vi "Get Caraya Library Information.vi"() -> (1 "Library Info":T1, 2 "Caraya Library Path":path, 3 "reserved":refnum<class>)   [LabVIEW 2013, in "Caraya.lvlib"]
uses:
  Caraya.lvlib
  Caraya Library Info.ctl
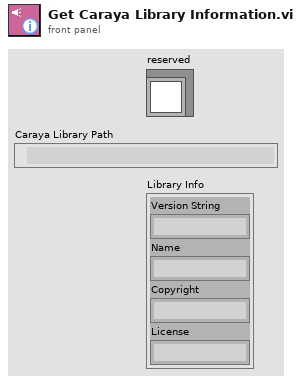
[diagram p1: front panel]
types:
  T1 = typedef "Caraya.lvlib/Caraya Library Info.ctl" = cluster{"Version String":string, "Name":string, "Copyright":string, "License":string}
  T2 = cluster{"Version String":string, "Name":string, "Copyright":string, "License":string}
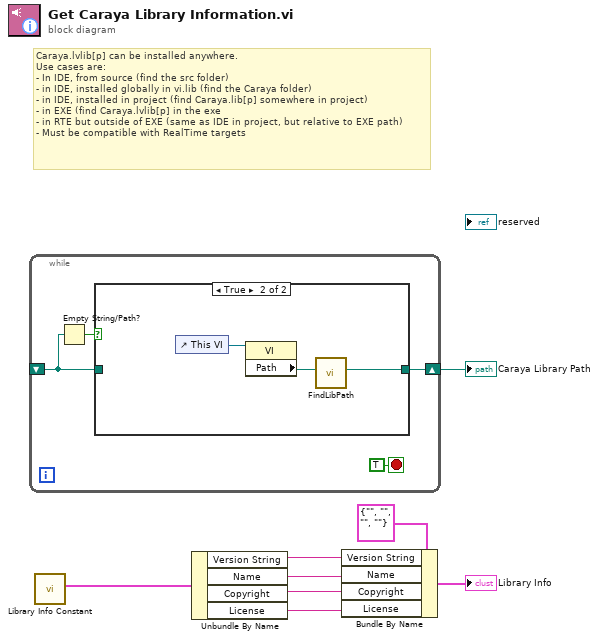
[diagram p0: block diagram]
diagram:
  # "Caraya.lvlib[p] can be installed anywhere.\nUse cases are: \n- In IDE, from source (find the src folder)\n- in IDE, installed globally in vi.lib (find the Caraya folder)\n- in IDE, installed in project (find Caraya.lib[p] somewhere in project)\n- in EXE (find Caraya.lvlib[p] in the exe\n- in RTE but outside of EXE (same as IDE in project, but relative to EXE path)\n- Must be compatible with RealTime targets"
  n1 = while {
    shift-right: [w12] -> w1
    shift-left: _ -> [w9]
    stop <- TRUE stop-if-true
    n2 = Empty String/Path?(string/path=w9) -> (empty?=w10:bool)
    n3 = case shown="True" w10 {
      tunnel: [w13 w16] -> w12
      tunnel: w9 -> [w13 _]
      frame False {
      }
      frame True {
        n4 = control-ref of="This VI"() -> (w15:refnum<vi>)
        n5 = property class="VI"(reference=w15) -> ("Path"=w14:path)  [unwired: 1 in, 2 out]
        n6 = call "FindLibPath.vi"("Caraya Library Member Path"=w14) -> ("Caraya Library Path"=w16:path)  [unwired: 10 in]
      }
    }
  }
  "Caraya Library Path" <- w1
  n7 = call "Library Info Constant.vi"() -> ("Library Info Constant"=w8:T2)  [unwired: 11 in]
  n8 = Unbundle By Name(w8) -> ("Version String"=w6:string, "Name"=w5:string, "Copyright"=w4:string, "License"=w3:string)
  n9 = Bundle By Name(cluster=T1 {"Version String"="", "Name"="", "Copyright"="", "License"=""} ("Caraya Library Info"), "Version String"=w6, "Name"=w5, "Copyright"=w4, "License"=w3) -> (→"Library Info":T1)
